vi "TimePlotAnnotations.vi"(7 "Top Plot":refnum<vi>, 8 "Negative Min":dbl, 9 "Negative TimingPlotData":T1[](array[typedef]), 10 "Postitive Max":dbl, 11 "Positive TimingPlotData":T1[](array[typedef])) -> ()   [LabVIEW 2014]
doc: "At its core, this VI annotates the elements of the timing plot. It also varies the element's heights between a sequence of three heights, and switches inactive elements to grey."
uses:
  Controls/TimingPlotData.ctl
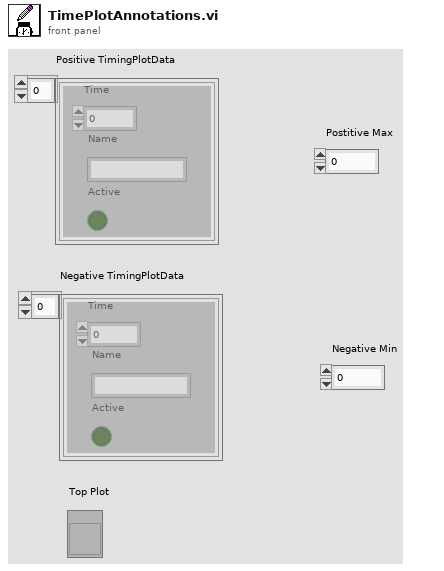
[diagram p1: front panel]
types:
  T1 = typedef "TimingPlotData.ctl" = cluster{"Time":dbl, "Name":string, "Active":bool}
  T2 = typedef "LVAnnotationListTypeDef.ctl" = cluster{"Name":string, "Color":u32, "Style":u8, "Point Style":u8, "Name Visible":bool, "Allow Drag":bool, "Annotation Mode":u32, "Plot":i32, "Index":i32, "Position":cluster{"X":dbl, "Y":dbl}, "X Scale":u32, "Y Scale":u32, "Show Arrow":bool, "Lock Name":bool, "Plot Area":i32, "Label Offset":cluster{"X":dbl, "Y":dbl}}[]
  T3 = cluster{"Name":string, "Color":u32, "Style":u8, "Point Style":u8, "Name Visible":bool, "Allow Drag":bool, "Annotation Mode":u32, "Plot":i32, "Index":i32, "Position":cluster{"X":dbl, "Y":dbl}, "X Scale":u32, "Y Scale":u32, "Show Arrow":bool, "Lock Name":bool, "Plot Area":i32, "Label Offset":cluster{"X":dbl, "Y":dbl}}
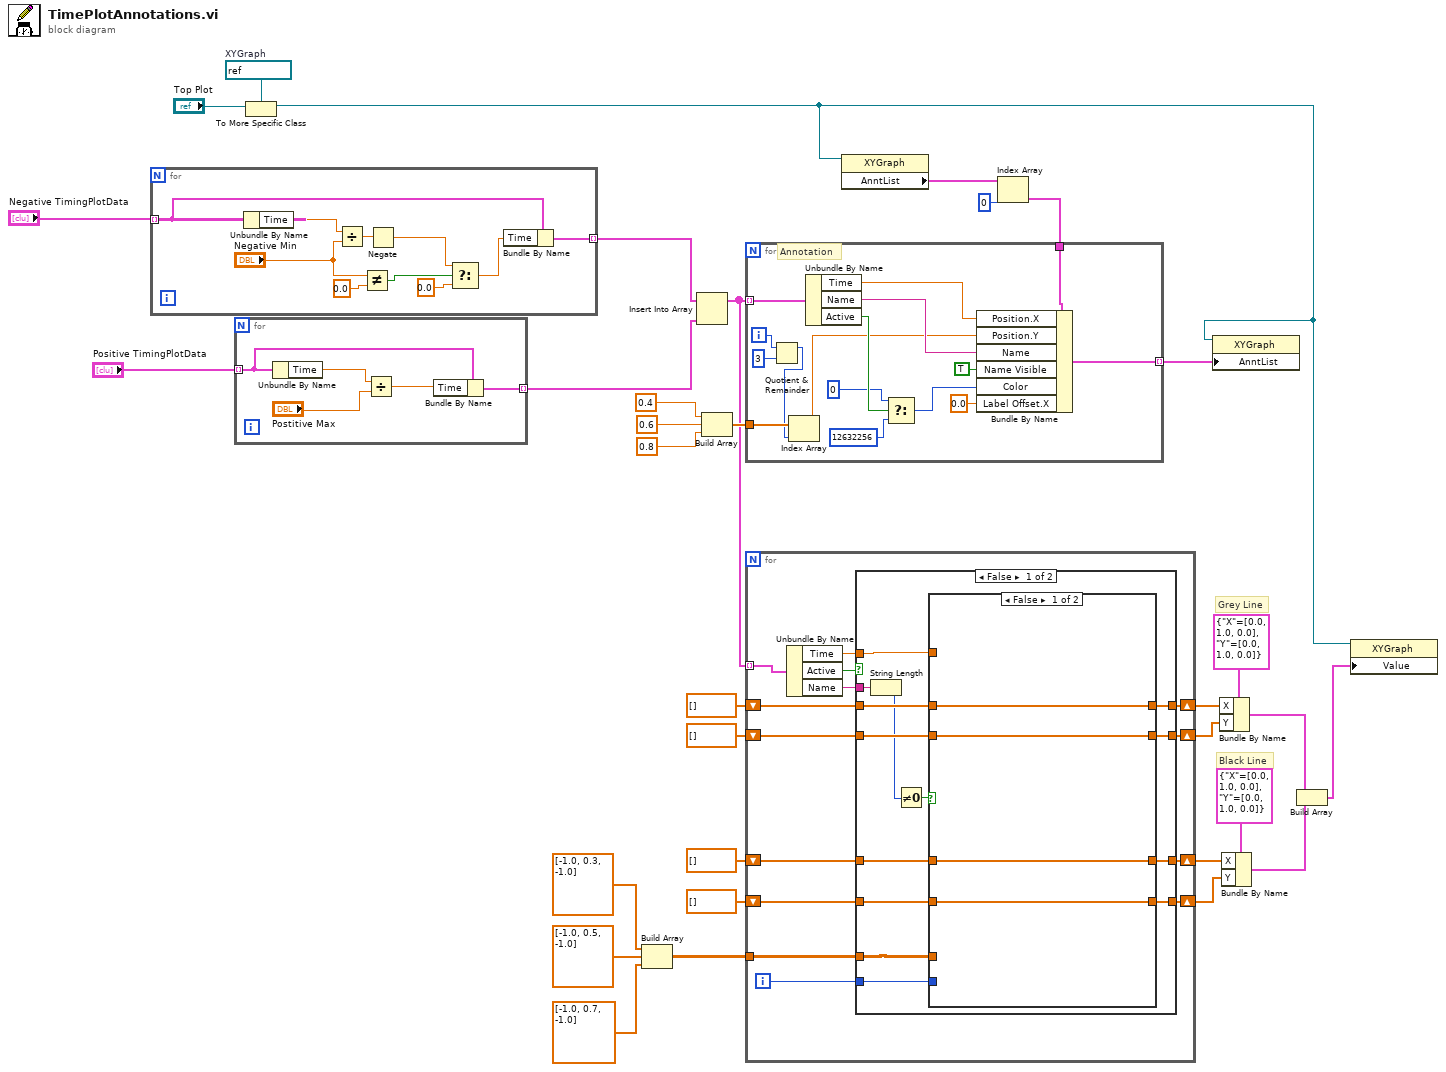
[diagram p0: block diagram]
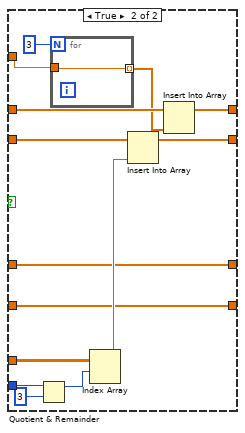
[diagram p2: hidden frame]
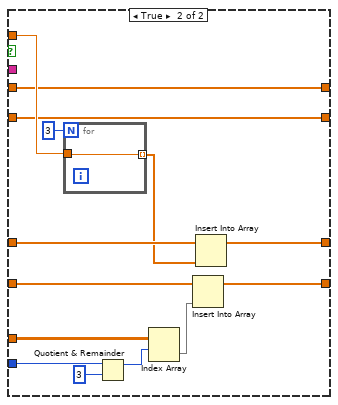
[diagram p3: hidden frame]
diagram:
  w20 = refnum<vi> refnum  # XYGraph
  # "Black Line"
  # "Grey Line"
  n1 = for {
    tunnel: "Negative TimingPlotData" -> [w41] mode=indexing
    tunnel: [w40] -> w31 mode=indexing
    n2 = Unbundle By Name(w41) -> ("Time"=w43:dbl)
    n3 = Divide(x=w43, y="Negative Min") -> (x/y=w42:dbl)
    n4 = Not Equal?(x="Negative Min", y=0.0) -> (x != y?=w38:bool)
    n5 = Negate(x=w42) -> (-x=w36:dbl)
    n6 = Select(t=w36, s=w38, f=0.0) -> (s? t:f=w35:dbl)
    n7 = Bundle By Name(cluster=w41, "Time"=w35) -> (w40:T1)
  }
  n8 = for {
    tunnel: "Positive TimingPlotData" -> [w47] mode=indexing
    tunnel: [w46] -> w30 mode=indexing
    n9 = Unbundle By Name(w47) -> ("Time"=w48:dbl)
    n10 = Divide(x=w48, y="Postitive Max") -> (x/y=w44:dbl)
    n11 = Bundle By Name(cluster=w47, "Time"=w44) -> (w46:T1)
  }
  n12 = To More Specific Class(target class=w20, reference="Top Plot") -> (specific class reference=w6:refnum<vi>)  [unwired: 1 in, 1 out]
  n13 = Build Array(dbl[] [-1.0, 0.3, -1.0], dbl[] [-1.0, 0.5, -1.0], dbl[] [-1.0, 0.7, -1.0]) -> (w1:dbl[][])
  n14 = Insert Into Array(array=w31, new element=w30) -> (w5:T1[])  [unwired: 1 in]
  n15 = Build Array(0.4, 0.6, 0.8) -> (w22:dbl[])
  n16 = for {
    tunnel: w5 -> [w62] mode=indexing
    shift-right: [w57] -> w14
    shift-left: dbl[] [] -> [w54]
    shift-right: [w56] -> w13
    shift-left: dbl[] [] -> [w55]
    shift-right: [w59] -> w17
    shift-left: dbl[] [] -> [w53]
    shift-right: [w58] -> w16
    shift-left: dbl[] [] -> [w52]
    tunnel: w1 -> [w50]
    i -> [w51]
    n17 = Unbundle By Name(w62) -> ("Time"=w61:dbl, "Active"=w60:bool, "Name"=w49:string)
    n18 = case shown="False" w60 {
      tunnel: w61 -> [w76 w108]
      tunnel: [w73 w102] -> w59
      tunnel: [w74 w101] -> w58
      tunnel: [w64 w106] -> w57
      tunnel: [w63 w104] -> w56
      tunnel: w55 -> [w66 w105]
      tunnel: w54 -> [w65 w107]
      tunnel: w53 -> [w72 w102]
      tunnel: w52 -> [w75 w101]
      tunnel: w51 -> [w70 w99]
      tunnel: w50 -> [w71 w97]
      tunnel: w49 -> [w69 _]
      frame False {
        n19 = String Length(string=w69) -> (length=w67:i32)
        n20 = Not Equal To 0?(x=w67) -> (x != 0?=w68:bool)
        n21 = case shown="False" w68 {
          tunnel: w76 -> [_ w93]
          tunnel: w75 -> [w79 w92]
          tunnel: [w79 w91] -> w74
          tunnel: [w80 w90] -> w73
          tunnel: w72 -> [w80 w89]
          tunnel: w71 -> [_ w85]
          tunnel: w70 -> [_ w84]
          tunnel: w66 -> [w78 w81]
          tunnel: w65 -> [w77 w82]
          tunnel: [w77 w82] -> w64
          tunnel: [w78 w81] -> w63
          frame False {
          }
          frame True {
            n22 = Quotient & Remainder(x=w84, y=3) -> (x-y*floor(x/y)=w86:i32)  [unwired: 1 out]
            n23 = for {
              N: 3 -> [_]
              tunnel: [w95] -> w88 mode=indexing
              tunnel: w93 -> [w95]
            }
            n24 = Index Array(array=w85, index (row)=w86) -> (element=w83:dbl[])  [unwired: 1 in]
            n25 = Insert Into Array(array=w92, new element=w83) -> (w91:dbl[])  [unwired: 1 in]
            n26 = Insert Into Array(array=w89, new element=w88) -> (w90:dbl[])  [unwired: 1 in]
          }
        }
      }
      frame True {
        n27 = for {
          N: 3 -> [_]
          tunnel: [w110] -> w103 mode=indexing
          tunnel: w108 -> [w110]
        }
        n28 = Quotient & Remainder(x=w99, y=3) -> (x-y*floor(x/y)=w100:i32)  [unwired: 1 out]
        n29 = Index Array(array=w97, index (row)=w100) -> (element=w96:dbl[])  [unwired: 1 in]
        n30 = Insert Into Array(array=w107, new element=w96) -> (w106:dbl[])  [unwired: 1 in]
        n31 = Insert Into Array(array=w105, new element=w103) -> (w104:dbl[])  [unwired: 1 in]
      }
    }
  }
  n32 = property class="XYGraph"(reference=w6) -> ("AnntList"=w29:T2)  [unwired: 1 in, 2 out]
  n33 = Index Array(array=w29, index=0) -> (element=w27:T3)
  n34 = for {
    tunnel: w27 -> [w126]
    tunnel: [w124] -> w26 mode=indexing
    tunnel: w5 -> [w123] mode=indexing
    tunnel: w22 -> [w114]
    i -> [w116]
    # "Annotation"
    n35 = Quotient & Remainder(x=w116, y=3) -> (x-y*floor(x/y)=w113:i32)  [unwired: 1 out]
    n36 = Index Array(array=w114, index=w113) -> (element=w112:dbl)
    n37 = Unbundle By Name(w123) -> ("Time"=w122:dbl, "Name"=w121:string, "Active"=w120:bool)
    n38 = Select(t=u32 0, s=w120, f=u32 12632256 ("Color")) -> (s? t:f=w117:u32)
    n39 = Bundle By Name(cluster=w126, "Position.X"=w122, "Position.Y"=w112, "Name"=w121, "Name Visible"=TRUE, "Color"=w117, "Label Offset.X"=0.0) -> (w124:T3)
  }
  n40 = property class="XYGraph"(reference=w6, "AnntList"=w26) -> ()  [unwired: 1 in, 2 out]
  n41 = Bundle By Name(cluster=cluster{"X":dbl[], "Y":dbl[]} {"X"=[0.0, 1.0, 0.0], "Y"=[0.0, 1.0, 0.0]}, "X"=w17, "Y"=w16) -> (w7:cluster{"X":dbl[], "Y":dbl[]})
  n42 = Bundle By Name(cluster=cluster{"X":dbl[], "Y":dbl[]} {"X"=[0.0, 1.0, 0.0], "Y"=[0.0, 1.0, 0.0]}, "X"=w13, "Y"=w14) -> (w8:cluster{"X":dbl[], "Y":dbl[]})
  n43 = Build Array(w8, w7) -> (w19:cluster{"X":dbl[], "Y":dbl[]}[])
  n44 = property class="XYGraph"(reference=w6, "Value"=w19) -> ()  [unwired: 1 in, 2 out]
